vi "Beta 2.0.2.vi"() -> ()   [LabVIEW 2011]
uses:
  <vilib>/vision/NI_Vision_Development_Module.lvlib
panel:
  out "Grayscale":T1(plugin-control)
  in  "Stop":bool
  in  "Browse":bool
  out "XY Graph":cluster{dbl[], dbl[]}(graph)
  out "Original Image":T1(plugin-control)
  out "Path to Image":path
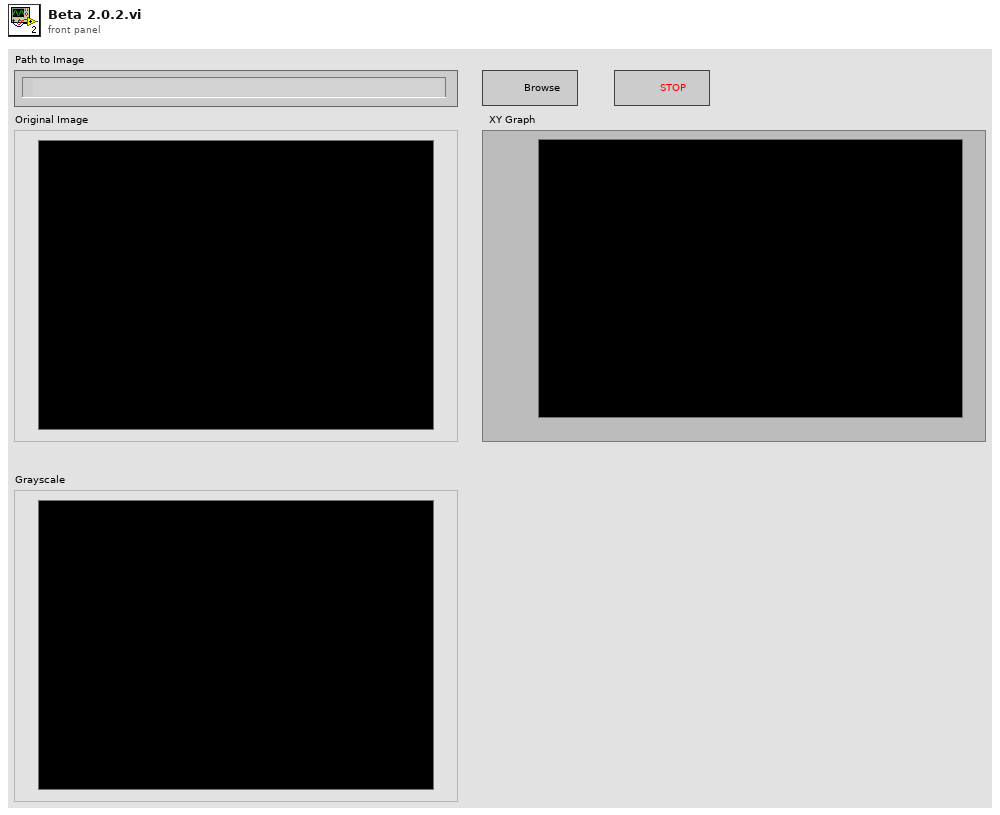
[diagram p1: front panel]
types:
  T1 = typedef "IMAQ Image.ctl" = refnum<image>
  T2 = typedef "Image Type" = u32
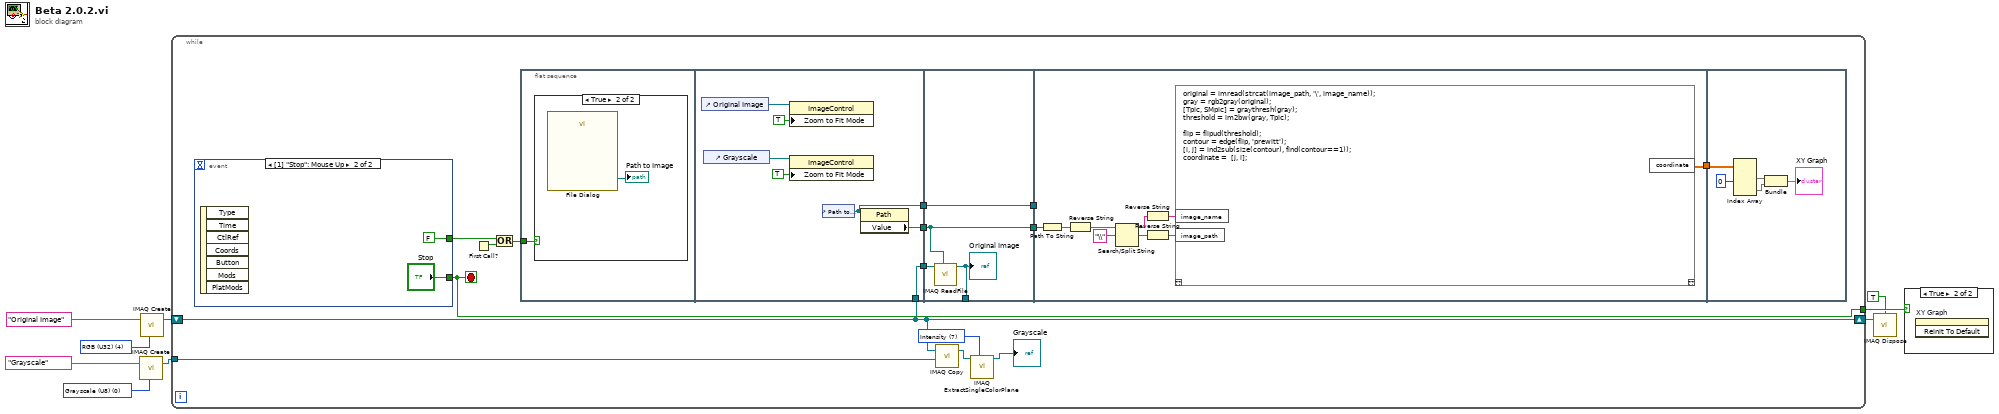
[diagram p0: block diagram]
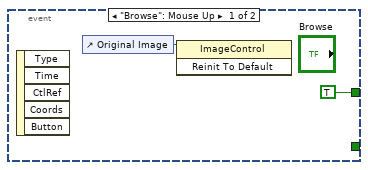
[diagram p3: hidden frame]
diagram:
  w3 = T2 0 items=["Grayscale (U8)", "Grayscale (I16)", "Grayscale (SGL)", "Complex (CSG)", "RGB (U32)", "HSL (U32)", "RGB (U64)", "Grayscale (U16)"] ("Image Type")
  w8 = T2 4 items=["Grayscale (U8)", "Grayscale (I16)", "Grayscale (SGL)", "Complex (CSG)", "RGB (U32)", "HSL (U32)", "RGB (U64)", "Grayscale (U16)"] ("Image Type")
  n1 = call "IMAQ Create"("Image Name"="Grayscale", "Image Type"=w3) -> ("New Image"=w2:T1)  [unwired: 3 in, 1 out]
  n2 = call "IMAQ Create"("Image Name"="Original Image", "Image Type"=w8) -> ("New Image"=w7:T1)  [unwired: 3 in, 1 out]
  n3 = while {
    shift-right: [w13] -> w6
    shift-left: w7 -> [w13]
    tunnel: [w15] -> w5
    tunnel: w2 -> [w14]
    stop <- w15 stop-if-true
    w10 = 7 items=["Red", "Green", "Blue", "Hue", "Saturation", "Luminance", "Value", "Intensity"] ("Color Plane")
    n4 = event shown="[1] \"Stop\": Mouse Up" {
      selector: _ -> [_ _]
      dyn-events: _ -> [_ _]
      timeout: _ -> [_ _]
      tunnel: [TRUE FALSE] -> w21
      tunnel: [_ "Stop"] -> w15
      event "Browse": Mouse Up {
        n5 = event-data() -> ()  [unwired: 1 in, 5 out]
        n6 = control-ref of="Original Image"() -> (w26:refnum<vi>)
        n7 = invoke class="ImageControl" method="Reinit To Default"(reference=w26) -> ()  [unwired: 2 in, 3 out]
      }
      event "Stop": Mouse Up {
        n8 = event-data() -> ()  [unwired: 1 in, 7 out]
      }
    }
    n9 = First Call?() -> (First Call?: T/F=w19:bool)
    n10 = Or(x=w21, y=w19) -> (x .or. y?=w18:bool)
    n11 = flat-sequence {
      tunnel: w18 -> [w29]
      tunnel: [w33] -> w22
      tunnel: [w35] -> w20
      tunnel: [w34] -> w17
      tunnel: w13 -> [w33]
      tunnel: [w39] -> w24
      tunnel: [w41] -> _
      tunnel: w22 -> [w40]
      tunnel: w20 -> [w39]
      tunnel: w17 -> [w38]
      tunnel: [w38] -> w16
      tunnel: w24 -> [_]
      tunnel: [w43] -> w23
      tunnel: w16 -> [w42]
      tunnel: w23 -> [w55]
      frame #0 {
        n12 = case shown="True" w29 {
          frame False {
          }
          frame True {
            n13 = call "File Dialog"() -> ("selected path"=→"Path to Image":path)  [unwired: 12 in, 3 out]
          }
        }
      }
      frame #1 {
        n14 = control-ref of="Original Image"() -> (w37:refnum<vi>)
        n15 = control-ref of="Grayscale"() -> (w31:refnum<vi>)
        n16 = property class="ImageControl"(reference=w37, "Zoom to Fit Mode"=TRUE) -> ()  [unwired: 1 in, 2 out]
        n17 = property class="ImageControl"(reference=w31, "Zoom to Fit Mode"=TRUE) -> ()  [unwired: 1 in, 2 out]
        n18 = control-ref of="Path to Image"() -> (w35:refnum<vi>)
        n19 = property class="Path"(reference=w35) -> ("Value"=w34:path)  [unwired: 1 in, 2 out]
      }
      frame #2 {
        n20 = call "IMAQ ReadFile"("File Path"=w38, "Image"=w40) -> ("Image Out"=w41:T1)  [unwired: 5 in, 4 out]
        "Original Image" <- w41
      }
      frame #3 {
        n21 = Path To String(path=w42) -> (string=w50:string)
        n22 = Reverse String(1:w50) -> (0:w49:string)
        n23 = Search/Split String(string=w49, search string/char (-)="\\") -> (substring before match=w47:string, match + rest of string=w46:string)  [unwired: 1 in, 1 out]
        n24 = Reverse String(1:w47) -> (0:w45:string)
        n25 = Reverse String(1:w46) -> (0:w44:string)
        n26 = script code="original = imread(strcat(image_path, '\\', image_name));\ngray = rgb2gray(original);\n[Tpic, SMpic] = graythresh(gray);\nthreshold = im2bw(gray, Tpic);\n\nflip = flipud(threshold);\ncontour = edge(flip, 'prewitt');\n[i, j] = ind2sub(size(contour), find(contour==1));\ncoordinate =  [j, i];"("image_name"=w45, "image_path"=w44) -> ("coordinate"=w43:dbl[][])  [unwired: 1 in, 1 out]
      }
      frame #4 {
        n27 = Index Array(array=w55, index (col) #1=0 ("disabled index (col)")) -> (element #1=w53:dbl[], element #2=w52:dbl[])  [unwired: 3 in]
        n28 = Bundle(w53, w52) -> (→"XY Graph":cluster{dbl[], dbl[]})  [unwired: 1 in]
      }
    }
    n29 = call "IMAQ Copy"("Image Dst"=w14, "Image Src"=w13) -> ("Image Dst Out"=w12:T1)  [unwired: 4 in, 1 out]
    n30 = call "IMAQ ExtractSingleColorPlane"("Color Plane"=w10, "Image Src"=w12) -> ("Image Dst Out"=→"Grayscale":T1)  [unwired: 8 in, 1 out]
  }
  n31 = call "IMAQ Dispose"("All Images? (No)"=TRUE, "Image"=w6) -> ()  [unwired: 4 in, 1 out]
  n32 = case shown="True" w5 {
    frame False {
    }
    frame True {
      n33 = invoke on="XY Graph" class="XYGraph (strict)" method="Reinit To Default"() -> ()  [unwired: 3 in, 3 out]
    }
  }
